vi "InitRollers.vi"() -> (0 "error out":errorcluster, 2 "Top Roller":T1, 3 "Bottom Roller":T1)   [LabVIEW 2015]
uses:
  Framework/Detailed Motor Type Def.ctl
  <vilib>/Rock Robotics/WPI/MotorControl/WPI_MotorControlDeviceRef.ctl
  <vilib>/Rock Robotics/WPI/MotorControl/WPI_MotorControlType.ctl
  <vilib>/Rock Robotics/SystemInterfaces/DIO/FPGA_DIOPWMChannel.ctl
  <vilib>/Rock Robotics/WPI/PWM/WPI_PWMDeadband.ctl
  <vilib>/Rock Robotics/WPI/CAN/Jaguar/SubVIs/WPI_CANJaguar_ControlMode.ctl
  <vilib>/Rock Robotics/WPI/CAN/TalonSRX/WPI_CANTalonSRX_APIControlMode.ctl
  <vilib>/Rock Robotics/WPI/MotorControl/WPI_MotorControlOpenCANTalonSRX.vi
  Shooter Global.vi
panel:
  in  "Detaled Motor Type Def in":T1
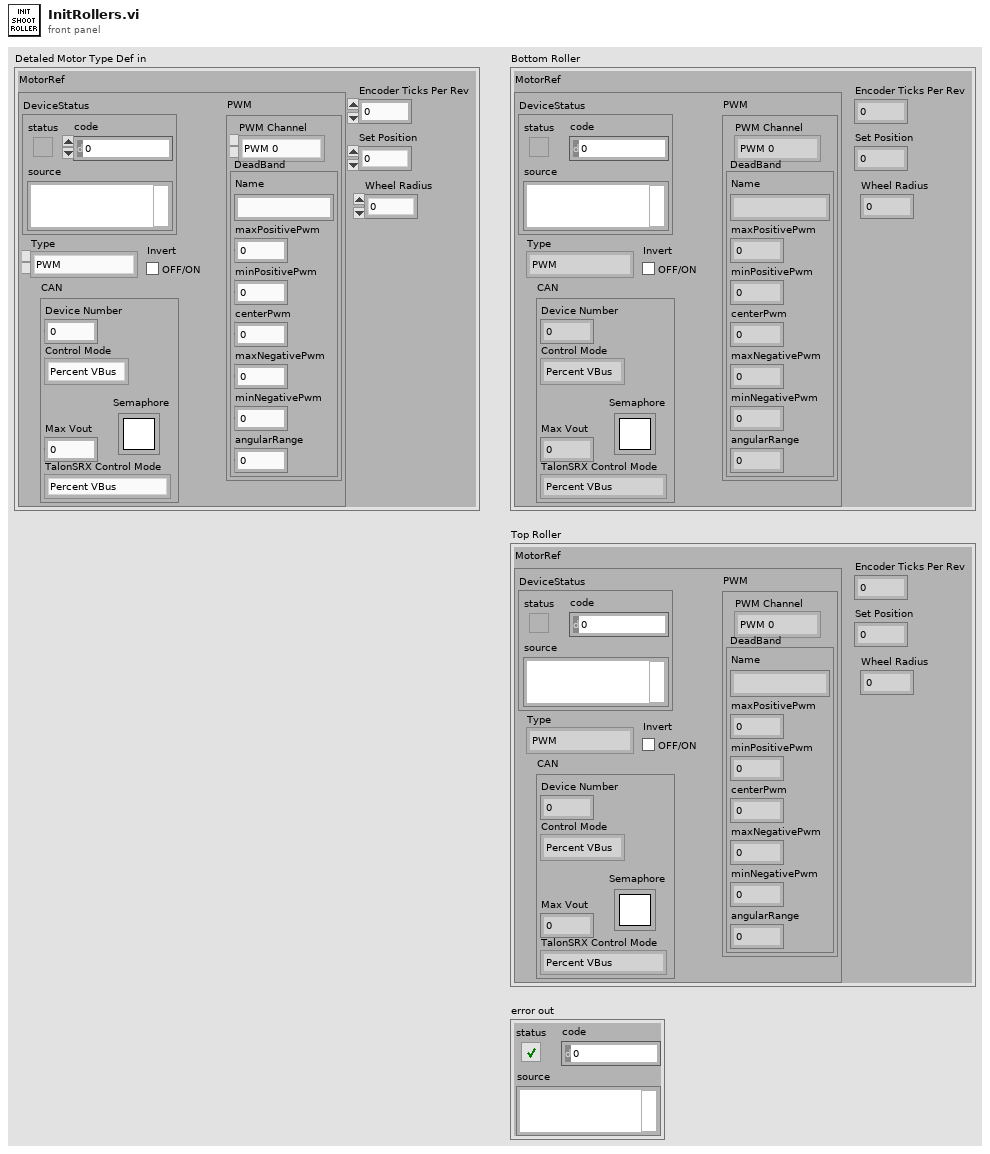
[diagram p1: front panel]
types:
  T1 = typedef "Detailed Motor Type Def.ctl" = cluster{"MotorRef":T2, "Encoder Ticks Per Rev":dbl, "Set Position":dbl, "Wheel Radius":dbl}
  T2 = typedef "WPI_MotorControlDeviceRef.ctl" = cluster{"DeviceStatus":errorcluster, "Type":T3, "PWM":cluster{"PWM Channel":T4, "DeadBand":T5}, "CAN":cluster{"Device Number":u8, "Control Mode":T6, "Semaphore":T7, "Max Vout":dbl, "TalonSRX Control Mode":T8}, "Invert":bool}
  T3 = typedef "WPI_MotorControlType.ctl" = enum16{"PWM", "CAN", "CANTalonSRX"}
  T4 = typedef "FPGA_DIOPWMChannel.ctl" = enum8{"PWM 0", "PWM 1", "PWM 2", "PWM 3", "PWM 4", "PWM 5", "PWM 6", "PWM 7", "PWM 8", "PWM 9", "PWM MXP 0", "PWM MXP 1", "PWM MXP 2", "PWM MXP 3", "PWM MXP 4", "PWM MXP 5", "PWM MXP 6", "PWM MXP 7", "PWM MXP 8", "PWM MXP 9", "Invalid"}
  T5 = typedef "WPI_PWMDeadband.ctl" = cluster{"Name":string, "maxPositivePwm":i32, "minPositivePwm":i32, "centerPwm":i32, "maxNegativePwm":i32, "minNegativePwm":i32, "angularRange":u16}
  T6 = typedef "WPI_CANJaguar_ControlMode.ctl" = enum8{"Percent VBus", "Current", "Speed", "Position", "Voltage"}
  T7 = typedef "Semaphore RefNum" = refnum<k1>
  T8 = typedef "WPI_CANTalonSRX_APIControlMode.ctl" = enum8{"Percent VBus", "Speed", "Position", "Slave", "Unchanged / Invalid", "Voltage Compensation", "Current", "Motion Profile"}
  T9 = cluster{"Top Roller":errorcluster, "Bottom Roller":errorcluster}
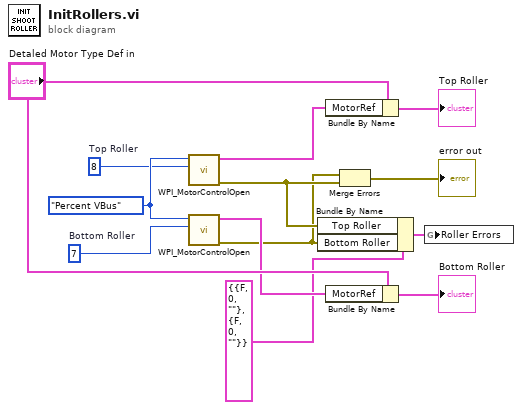
[diagram p0: block diagram]
diagram:
  w6 = u8 8  # Top Roller
  w5 = u8 7  # Bottom Roller
  w11 = WPI_CANTalonSRX_APIControlMode."Percent VBus" ("Control Mode")
  n1 = call-poly <vilib>:"WPI_MotorControlOpen.vi"("Device Number"=w6, "Control Mode"=w11) -> ("error out"=w2:errorcluster, "MotorControlDeviceRef"=w9:T2)  [unwired: 8 in]
  n2 = call-poly <vilib>:"WPI_MotorControlOpen.vi"("Device Number"=w5, "Control Mode"=w11) -> ("error out"=w1:errorcluster, "MotorControlDeviceRef"=w7:T2)  [unwired: 8 in]
  n3 = Bundle By Name(cluster=T9 {"Top Roller"={"status"=FALSE, "code"=0, "source"=""}, "Bottom Roller"={"status"=FALSE, "code"=0, "source"=""}} ("Roller Errors"), "Top Roller"=w2, "Bottom Roller"=w1) -> (w4:T9)
  n4 = Bundle By Name(cluster="Detaled Motor Type Def in", "MotorRef"=w9) -> (→"Top Roller":T1)
  n5 = Bundle By Name(cluster="Detaled Motor Type Def in", "MotorRef"=w7) -> (→"Bottom Roller":T1)
  n6 = Merge Errors(w1, w2) -> (→"error out":errorcluster)
  n7 = global write "Shooter Global.vi" "Roller Errors"(w4) -> ()
